vi "event_record.vi"(4 "record":refnum<vi>, 5 "Event Data":cluster{"record":variant}, 6 "Control Ref":refnum<k7>, 7 "Event Common Data":T1) -> ()   [LabVIEW 2011]
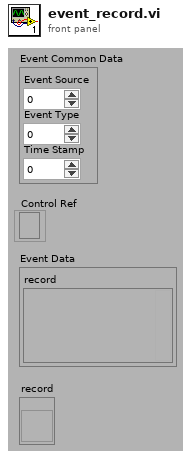
[diagram p1: front panel]
types:
  T1 = cluster{"Event Source":i32, "Event Type":u32, "Time Stamp":u32}
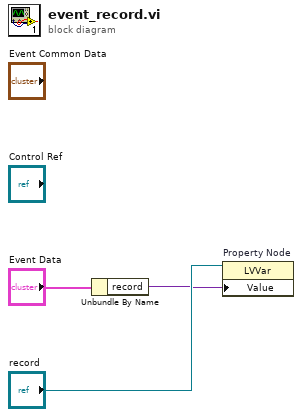
[diagram p0: block diagram]
diagram:
  n1 = Unbundle By Name "Unbundle By Name"("Event Data") -> ("record"=w1:variant)
  n2 = property on="Property Node" class="LVVar"(reference="record", "Value"=w1) -> ()  [unwired: 1 in, 2 out]
